vi "Configure Connection.vi"(8 "error in (no error)":errorcluster, 11 "BLE context in":refnum<class "BLE context.lvclass">) -> (0 "error out":errorcluster, 3 "BLE context out":refnum<class "BLE context.lvclass">, 5 "Device name":string)   [LabVIEW 2015, in "BLE context.lvclass"]
uses:
  BLE context.lvclass
  BLE context.lvclass/BLE context.ctl
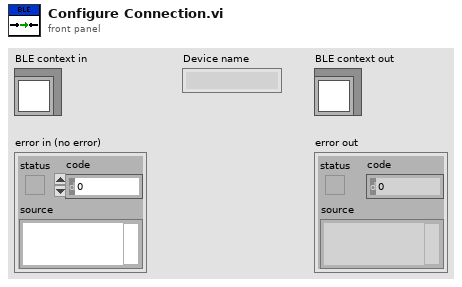
[diagram p1: front panel]
types:
  T1 = typedef "connection_status_bundle.ctl" = cluster{"MAC Address":string, "cnx handle":u8, "cnx flags":u8, "Address Type":T2, "Connection Interval (ms)":u16, "Timeout(ms)":u16, "Latency":u16, "bonding handle":u8}
  T2 = typedef "address_type.ctl" = u8
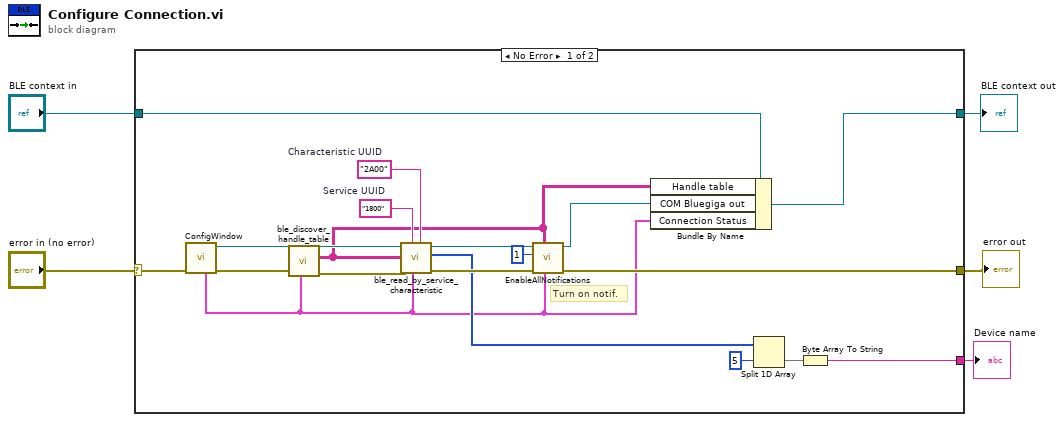
[diagram p0: block diagram]
diagram:
  n1 = case shown="No Error" "error in (no error)" {
    selector: "error in (no error)" -> [w18 w27]
    tunnel: [w13 w27] -> w4
    tunnel: [w16 w26] -> w2
    tunnel: "BLE context in" -> [w17 w26]
    tunnel: [w9 _] -> w1
    frame No Error {
      w22 = "2A00"  # Characteristic UUID
      w23 = "1800"  # Service UUID
      # "Turn on notif."
      n2 = call "ConfigWindow.vi"("error in"=w18) -> ("error out"=w8:errorcluster, "COM Bluegiga out"=w6:refnum<visa-resource-name>, "Connection Status"=w7:T1)  [unwired: 8 in]
      n3 = call <vilib>:"ble_discover_handle_table.vi"("Connection Status"=w7, "error in (no error)"=w8, "COM Bluegiga in"=w6) -> ("error out"=w25:errorcluster, "Handle table"=w14:string[][], "COM Bluegiga out"=w24:refnum<visa-resource-name>)  [unwired: 6 in]
      n4 = call <vilib>:"ble_read_by_service_characteristic.vi"("Characteristic UUID"=w22, "Connection Status"=w7, "Service UUID"=w23, "error in (no error)"=w25, "Handle table"=w14, "COM Bluegiga in"=w24) -> ("error out"=w21:errorcluster, "characteristic value"=w10:u8[], "COM Bluegiga out"=w20:refnum<visa-resource-name>)  [unwired: 3 in]
      n5 = call "EnableAllNotifications.vi"("Connection Status"=w7, "Handle table"=w14, "error in"=w21, "1 or 0"=u16 1, "COM Bluegiga in"=w20) -> ("error out"=w13:errorcluster, "COM Bluegiga out"=w15:refnum<visa-resource-name>)  [unwired: 5 in]
      n6 = Bundle By Name(cluster=w17, "Handle table"=w14, "COM Bluegiga out"=w15, "Connection Status"=w7) -> (w16:refnum<class "BLE context.lvclass">)
      n7 = Split 1D Array(array=w10, index=5) -> (second subarray=w11:u8[])  [unwired: 1 out]
      n8 = Byte Array To String(unsigned byte array=w11) -> (string=w9:string)
    }
    frame Error {
    }
  }
  "error out" <- w4
  "BLE context out" <- w2
  "Device name" <- w1
